vi "Update World.vi"(11 "Main Controller Actor in":refnum<class "Main Controller Actor.lvclass">) -> (3 "Main Controller Actor out":refnum<class "Main Controller Actor.lvclass">)   [LabVIEW 2015, in "Main Controller Actor.lvclass"]
uses:
  Main Controller Actor.lvclass
  Main Controller Actor.lvclass/Main Controller Actor.ctl
  Globals.vi
  Element/Element.lvclass
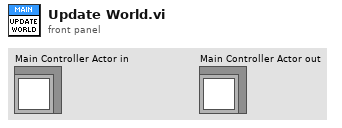
[diagram p1: front panel]
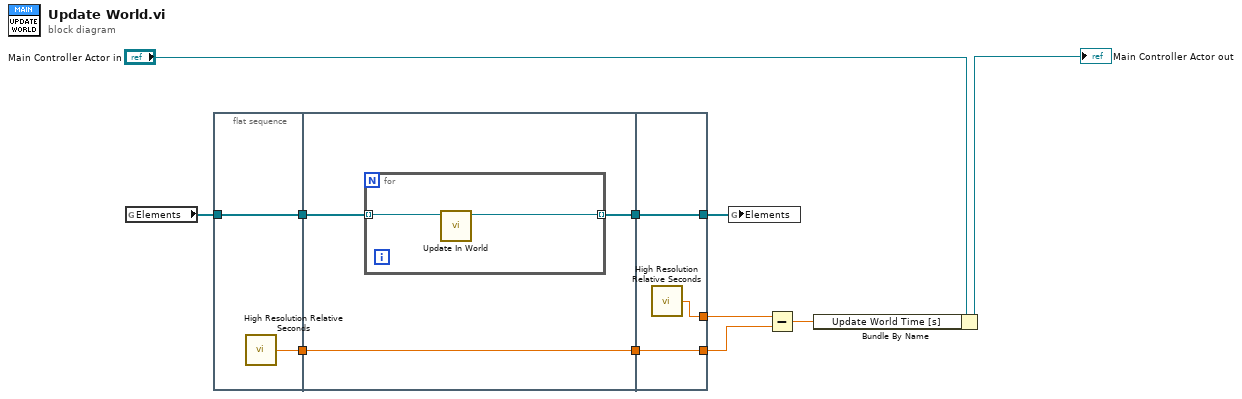
[diagram p0: block diagram]
diagram:
  n1 = global read "Globals.vi" "Elements"() -> (w10:refnum<class "Element.lvclass">[])
  n2 = flat-sequence {
    tunnel: w10 -> [w13]
    tunnel: [w13] -> w8
    tunnel: [w12] -> w7
    tunnel: [w16] -> w9
    tunnel: w8 -> [w15]
    tunnel: w7 -> [w14]
    tunnel: [w14] -> w6
    tunnel: [w21] -> w11
    tunnel: w9 -> [w21]
    tunnel: [w20] -> w4
    tunnel: w6 -> [w20]
    tunnel: [w19] -> w5
    frame #0 {
      n3 = call <vilib>:"High Resolution Relative Seconds.vi"() -> ("relative seconds"=w12:dbl)
    }
    frame #1 {
      n4 = for {
        tunnel: [w18] -> w16 mode=indexing
        tunnel: w15 -> [w17] mode=indexing
        n5 = call-dynamic "Update In World.vi"("Movable in"=w17) -> ("Movable out"=w18:refnum<class "Element.lvclass">)  [unwired: 10 in]
      }
    }
    frame #2 {
      n6 = call <vilib>:"High Resolution Relative Seconds.vi"() -> ("relative seconds"=w19:dbl)
    }
  }
  n7 = global write "Globals.vi" "Elements"(w11) -> ()
  n8 = Subtract(x=w5, y=w4) -> (x-y=w1:dbl)
  n9 = Bundle By Name(cluster="Main Controller Actor in", "Update World Time [s]"=w1) -> (→"Main Controller Actor out":refnum<class "Main Controller Actor.lvclass">)
